vi "Create CSI-2 Packet TDMS Files.vi"() -> ()   [LabVIEW 2025, in "GettingStarted_Gen_148X_Host.lvlib"]
uses:
  GettingStarted_Gen_148X_Host.lvlib
  Types/Frame Data Configuration.ctl
  <instrlib>/FlexRIO/CSI-2/v2/Common/Types/LLP Data Type.ctl
  Types/Frame Timing Configuration.ctl
  Common/GettingStarted_Common_148X_Host.lvlib
  <instrlib>/FlexRIO/CSI-2/v2/Common/NI CSI-2 API Common v2.lvlib
panel:
  out "Actrual Frame":i32
  in  "Generate LLP Packet Offsets":bool=TRUE
  in  "Serial Input Channels":string[](array[string])=["SI0"]
  out "Actual Frame Rate (fps)":dbl
  in  "Frame Timing Configuration":T1={"desired frame rate (fps)"=30.0, "actual link data rate (B/s)"=385000000.0, "minimum delay between packets (cycles)"=500, "line blanking (cycles)"=1000} {"actual link data rate (B/s)" format="%_6p"; "line blanking (cycles)" format="%#.0f"}
  in  "Number of Frames":i32=10
  in  "Frame Data Configuration":T2={"pixel data type"=enum."RAW 12", "horizontal resolution"=1920, "vertical resolution"=1080, "virtual channel"=0.0, "include line sync packets"=FALSE}
  out "Error Out":errorcluster
  in  "TDMS File Directory":path
  # "Overview: Create sample TDMS files for use with the Generation Getting Started example.  \nInstructions: Visit https://ni.com/r/automotive-camera-module-ref for a detailed tutorial or use the basic instructions below.\n\n 1. Select the serial input channel names to use when creating the files.  The Generation Getting Started example expects the serial input channel number of the file to match the serial output channel number used to generate the data.\n 2. Select the destination directory for the created TDMS files.  Leave blank to use the \"TDMS Files\" directory in the same directory as this VI.\n 3. Select the number of frames to create. \n 4. Select the frame data configuration.  This determines what the frames will look like.  Each frame will be identical with the exception of the frame number.  Each line within a frame will be identical with the exception of the line number (if configured to send line sync packets).  The packet payload is a byte ramp; this is independent of the pixel data type.\n 5. Select the frame timing configuration.  This determines the timing of the individual packets.  The Actual Frame Rate (fps) indicator shows the frame rate of the generated data.  It is possible that this will be lower than the desired frame rate because the interpacket delay cycles and line blanking cycles  are priortized over the frame rate."
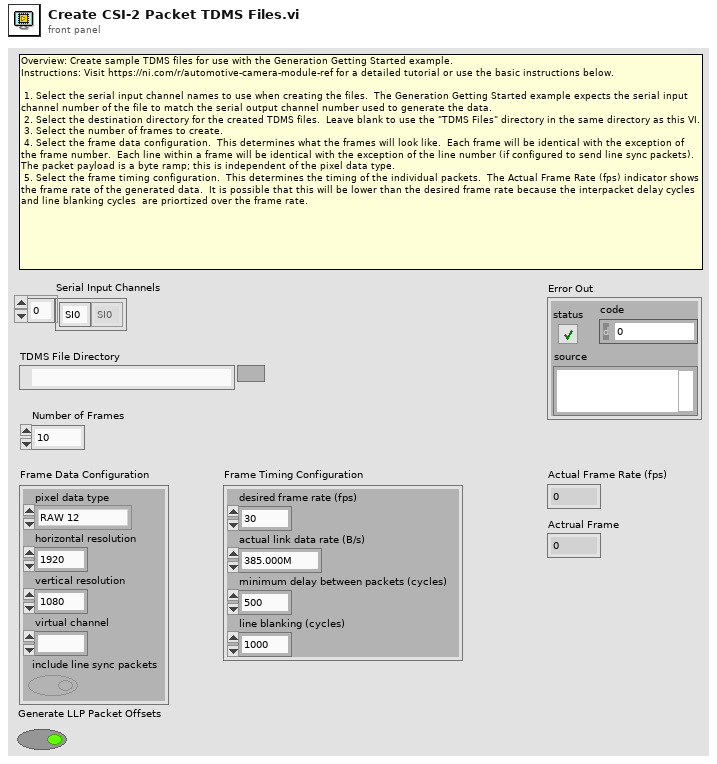
[diagram p1: front panel]
types:
  T1 = typedef "GettingStarted_Gen_148X_Host.lvlib/Frame Timing Configuration.ctl" = cluster{"desired frame rate (fps)":dbl, "actual link data rate (B/s)":dbl, "minimum delay between packets (cycles)":u64, "line blanking (cycles)":u64}
  T2 = typedef "GettingStarted_Gen_148X_Host.lvlib/Frame Data Configuration.ctl" = cluster{"pixel data type":T3, "horizontal resolution":u16, "vertical resolution":u16, "virtual channel":fxp<+,4,4>, "include line sync packets":bool}
  T3 = typedef "NI CSI-2 API Common v2.lvlib/LLP Data Type.ctl" = enum8{"Frame Start", "Frame End", "Line Start", "Line End", "End of Transmission", "Reserved 0", "Reserved 1", "Reserved 2", "Generic Short Packet 1", "Generic Short Packet 2", "Generic Short Packet 3", "Generic Short Packet 4", "Generic Short Packet 5", "Generic Short Packet 6", "Generic Short Packet 7", "Generic Short Packet 8", "Null", "Blanking Data", "Embedded 8-bit non Image Data", "Generic Long Packet 1", "Generic Long Packet 2", "Generic Long Packet 3", "Generic Long Packet 4", "Reserved 3", "YUV420 8-bit", "YUV420 10-bit", "Legacy YUV420 8-bit", "Reserved 4", "YUV420 8-bit Chroma Shifted", "YUV420 10-bit Chroma Shifted", "YUV422 8-bit", "YUV422 10-bit", "RGB444", "RGB555", "RGB565", "RGB666", "RGB888", "Reserved 5", "Reserved 6", "RAW 24", "RAW 6", "RAW 7", "RAW 8", "RAW 10", "RAW 12", "RAW 14", "RAW 16", "RAW 20", "User Defined 8-bit Data 1", "User Defined 8-bit Data 2", "User Defined 8-bit Data 3", "User Defined 8-bit Data 4", "User Defined 8-bit Data 5", "User Defined 8-bit Data 6", "User Defined 8-bit Data 7", "User Defined 8-bit Data 8", "USL Command", "Reserved 7", "Reserved 8", "Reserved 9", "Reserved 10", "Reserved 11", "Reserved 12", "LRTE EPD Spacer"}
  T4 = enum16{"open", "open or create", "create or replace", "create", "open (read-only)"}
  T5 = enum16{"big-endian, network order", "native, host order", "little-endian"}
  T6 = typedef "NI CSI-2 API Host v2.lvlib/Host LLP Packet.ctl" = cluster{"header":T7, "payload":u8[], "footer":T8}
  T7 = typedef "NI CSI-2 API FPGA v2.lvlib/LLP Packet Header.ctl" = cluster{"word count":u16, "ecc":fxp<+,6,6>, "vcx":fxp<+,2,2>, "data type":fxp<+,6,6>, "vc":fxp<+,2,2>}
  T8 = typedef "NI CSI-2 API FPGA v2.lvlib/LLP Packet Footer.ctl" = cluster{"crc":u16}
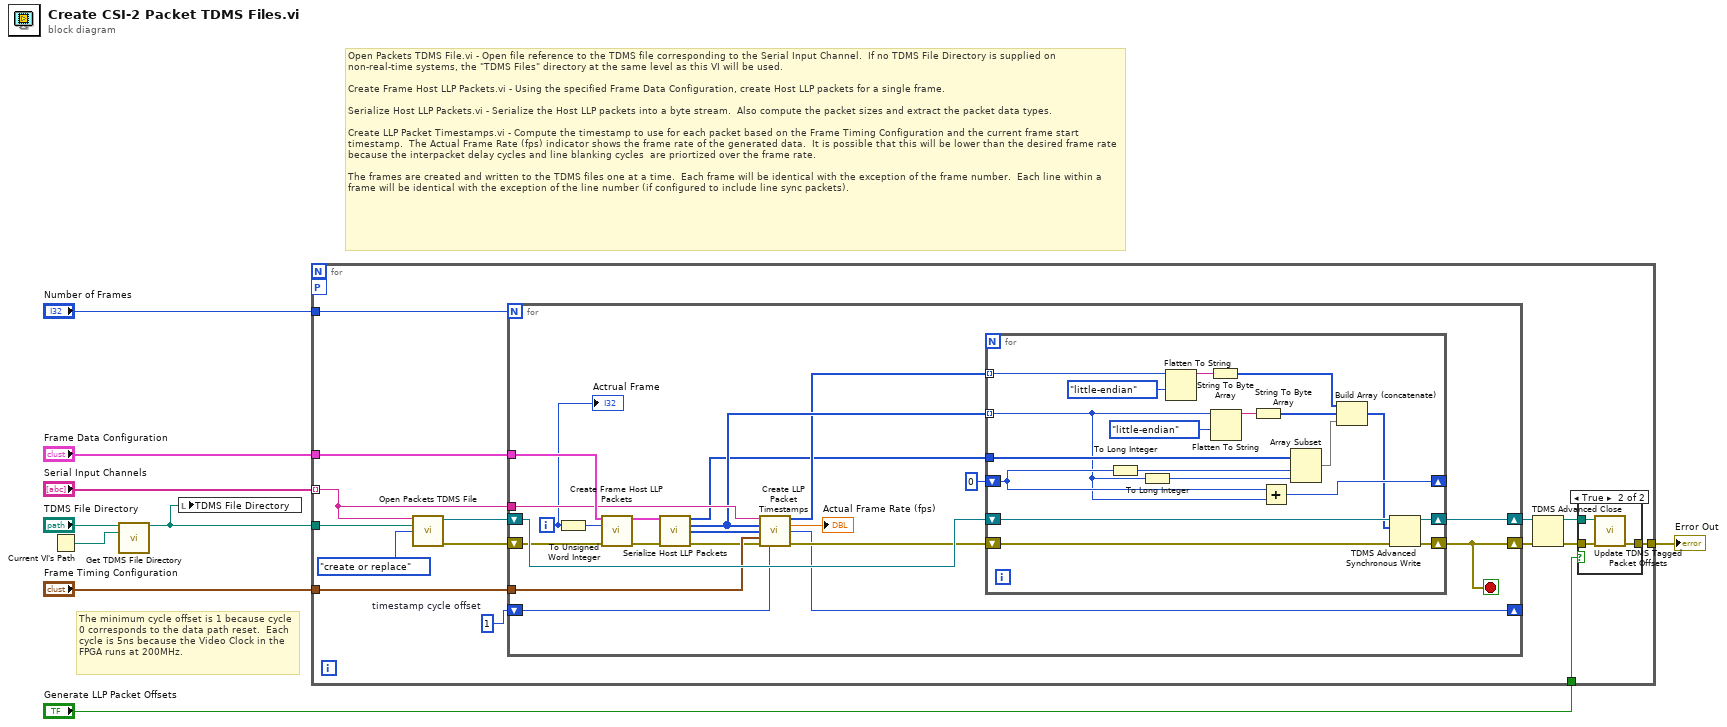
[diagram p0: block diagram]
diagram:
  # "The minimum cycle offset is 1 because cycle 0 corresponds to the data path reset.  Each cycle is 5ns because the Video Clock in the FPGA runs at 200MHz."
  # "Open Packets TDMS File.vi - Open file reference to the TDMS file corresponding to the Serial Input Channel.  If no TDMS File Directory is supplied on non-real-time systems, the \"TDMS Files\" directory at the same level as this VI will be used.\n\nCreate Frame Host LLP Packets.vi - Using the specified Frame Data Configuration, create Host LLP packets for a single frame.\n\nSerialize Host LLP Packets.vi - Serialize the Host LLP packets into a byte stream.  Also compute the packet sizes and extract the packet data types. \n\nCreate LLP Packet Timestamps.vi - Compute the timestamp to use for each packet based on the Frame Timing Configuration and the current frame start timestamp.  The Actual Frame Rate (fps) indicator shows the frame rate of the generated data.  It is possible that this will be lower than the desired frame rate because the interpacket delay cycles and line blanking cycles  are priortized over the frame rate.\n\nThe frames are created and written to the TDMS files one at a time.  Each frame will be identical with the exception of the frame number.  Each line within a frame will be identical with the exception of the line number (if configured to include line sync packets)."
  n1 = Current VI's Path() -> (path=w3:path)
  n2 = call "Get TDMS File Directory.vi"("tdms file directory in"="TDMS File Directory", "calling vi path"=w3) -> ("tdms file directory out"=w5:path)  [unwired: 13 in]
  n3 = local write "TDMS File Directory"(w5) -> ()
  n4 = for {
    tunnel: [w11] -> w2
    tunnel: "Frame Data Configuration" -> [w24]
    tunnel: "Number of Frames" -> [w23]
    tunnel: "Frame Timing Configuration" -> [w22]
    tunnel: w5 -> [w17]
    tunnel: "Serial Input Channels" -> [w18] mode=indexing
    workers-P: _ -> [_]
    tunnel: "Generate LLP Packet Offsets" -> [w10]
    w19 = u64 1  # timestamp cycle offset
    n5 = call "Open Packets TDMS File.vi"("serial input channel"=w18, "base tdms file path"=w17, "file operation type"=T4."create or replace") -> ("packets file ref"=w20:refnum<k34>, "error out"=w16:errorcluster)  [unwired: 11 in]
    n6 = for {
      N: w23 -> [_]
      tunnel: w24 -> [w48]
      tunnel: w18 -> [w46]
      shift-right: [w33] -> w21
      shift-left: w20 -> [w49]
      shift-right: [w43] -> _
      shift-left: w19 -> [w41]
      tunnel: w22 -> [w40]
      shift-right: [w34] -> w14
      shift-left: w16 -> [w47]
      i -> [w29]
      stop <- w34 stop-if-true
      n7 = To Unsigned Word Integer(number=w29) -> (unsigned 16bit integer=w44:u16)
      n8 = call "Create Frame Host LLP Packets.vi"("frame configuration"=w48, "frame number"=w44, "error in (no error)"=w47) -> ("frame packets"=w39:T6[], "error out"=w38:errorcluster)  [unwired: 11 in]
      n9 = call "Serialize Host LLP Packets.vi"("host llp packets"=w39, "error in (no error)"=w38) -> ("packet bytes"=w31:u8[], "packet sizes"=w37:u32[], "packet data types"=w36:T3[], "error out"=w35:errorcluster)  [unwired: 10 in]
      n10 = call "Create LLP Packet Timestamps.vi"("serial input channel"=w46, "llp packet sizes"=w37, "packet data types"=w36, "frame timing configuration"=w40, "error in (no error)"=w35, "frame start timestamp"=w41) -> ("timestamps"=w32:u64[], "actual frame rate (fps)"=→"Actual Frame Rate (fps)":dbl, "next frame start timestamp"=w43:u64, "error out"=w45:errorcluster)  [unwired: 6 in]
      n11 = for {
        tunnel: w37 -> [w58] mode=indexing
        tunnel: w32 -> [w68] mode=indexing
        shift-right: [w52] -> w33
        shift-left: w49 -> [w53]
        shift-right: [w54] -> w34
        shift-left: w45 -> [w51]
        shift-right: [w65] -> _
        shift-left: u32 0 -> [w63]
        tunnel: w31 -> [w64]
        n12 = To Long Integer(number=w63) -> (32bit integer=w60:i32)
        n13 = To Long Integer(number=w58) -> (32bit integer=w59:i32)
        n14 = Flatten To String(anything=w68, byte order (0:big-endian, network order)=T5."little-endian") -> (data string=w67:string)  [unwired: 2 in, 2 out]
        n15 = String To Byte Array(string=w67) -> (unsigned byte array=w55:u8[])
        n16 = Flatten To String(anything=w58, byte order (0:big-endian, network order)=T5."little-endian") -> (data string=w66:string)  [unwired: 2 in, 2 out]
        n17 = String To Byte Array(string=w66) -> (unsigned byte array=w56:u8[])
        n18 = Add(x=w63, y=w58) -> (x+y=w65:u32)
        n19 = Array Subset(array=w64, index=w60, length=w59) -> (w57:u8[])
        n20 = Build Array (concatenate)(w55, w56, w57) -> (w50:u8[])
        n21 = TDMS Advanced Synchronous Write(8:w51, 10:w50, 11:w53) -> (0:w54:errorcluster, 3:w52:refnum<k34>)
      }
      "Actrual Frame" <- w29
    }
    n22 = TDMS Advanced Close(8:w14, 11:w21) -> (0:w12:errorcluster, 3:w13:path)  [unwired: 2 in]
    n23 = case shown="True" w10 {
      tunnel: w13 -> [_ w28]
      tunnel: w12 -> [w25 w27]
      tunnel: [w25 w26] -> w11
      frame False {
      }
      frame True {
        n24 = call "Update TDMS Tagged Packet Offsets.vi"("llp tagged packet file path"=w28, "error in"=w27) -> ("error out"=w26:errorcluster)  [unwired: 12 in, 1 out]
      }
    }
  }
  "Error Out" <- w2
